vi "Num2BoolArr.vi"(1 "Number of Booleans":i32, 2 "Number":u32) -> (0 "Boolean Array":bool[](array[boolean]))   [LabVIEW 2016, in "Common.lvlib"]
uses:
  <userlib>/Common Components/Common/Common.lvlib
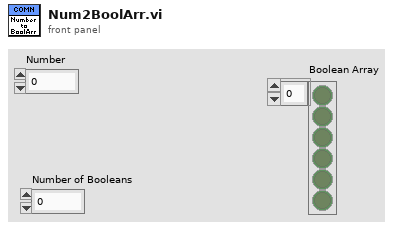
[diagram p1: front panel]
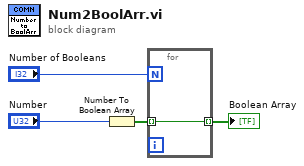
[diagram p0: block diagram]
diagram:
  n1 = Number To Boolean Array(number="Number") -> (Boolean array=w3:bool[])
  n2 = for {
    N: "Number of Booleans" -> [_]
    tunnel: w3 -> [w5] mode=indexing
    tunnel: [w5] -> w1 mode=indexing
  }
  "Boolean Array" <- w1
